vi "CRC-32.vi"(6 "Reflected":bool, 8 "FinalXorValue":u32 format="%08x", 9 "InitialCRC":u32 format="%08x", 10 "Polynomial":u32 format="%08x", 11 "DATA":u8[](array[numeric]) format="%02x") -> (3 "CRC":u32 format="%08x")   [LabVIEW 2021, in "LIN Frame Protection Addon Engine.lvlib"]
uses:
  LIN Frame Protection Addon Engine.lvlib
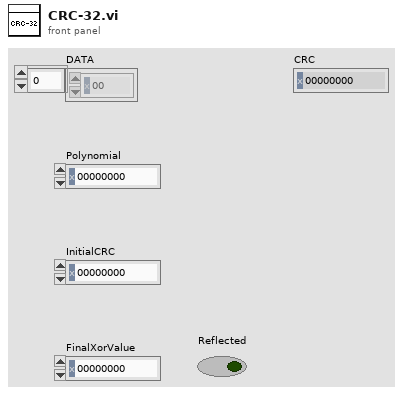
[diagram p1: front panel]
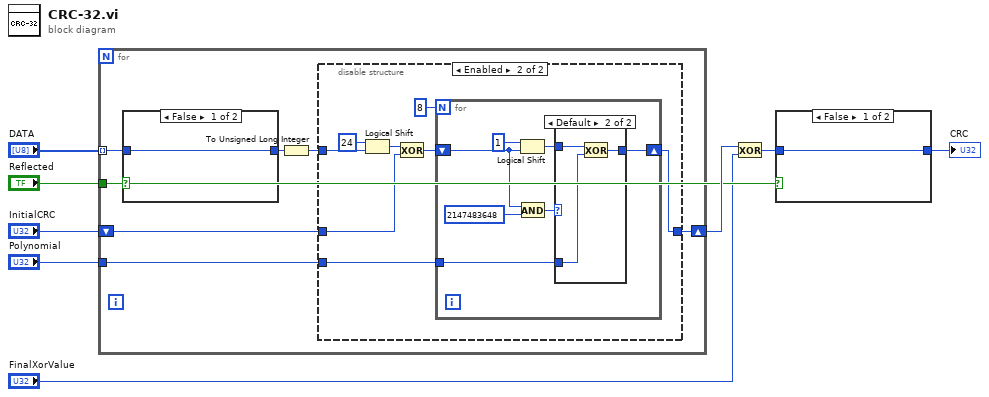
[diagram p0: block diagram]
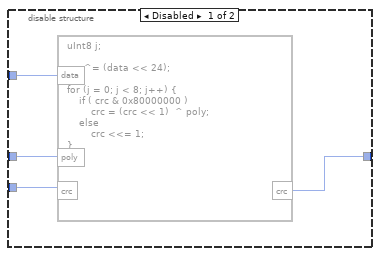
[diagram p2: hidden frame]
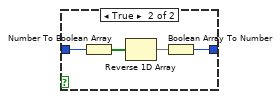
[diagram p4: hidden frame]
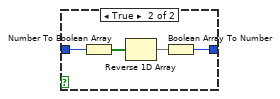
[diagram p5: hidden frame]
diagram:
  n1 = for {
    tunnel: "Polynomial" -> [w15]
    tunnel: "DATA" -> [w13] mode=indexing
    tunnel: "Reflected" -> [w14]
    shift-right: [w10] -> w6
    shift-left: "InitialCRC" -> [w11]
    n2 = case shown="False" w14 {
      tunnel: [w39 w42] -> w12
      tunnel: w13 -> [w39 w43]
      frame False {
      }
      frame True {
        n3 = Number To Boolean Array(number=w43) -> (Boolean array=w41:bool[])
        n4 = Reverse 1D Array(array=w41) -> (reversed array=w40:bool[])
        n5 = Boolean Array To Number(Boolean array=w40) -> (number=w42:u8)
      }
    }
    n6 = To Unsigned Long Integer(number=w12) -> (unsigned 32bit integer=w9:u32)
    n7 = disable-structure shown="Enabled" {
      disable-tunnel: w15 -> [w19 w22]
      disable-tunnel: w9 -> [w18 w27]
      disable-tunnel: w11 -> [w17 w25]
      disable-tunnel: [w16 w21] -> w10
      frame Disabled {
        n8 = formula code="uInt8 j;\n\ncrc ^= (data << 24);\n\nfor (j = 0; j < 8; j++) {\n    if ( crc & 0x80000000 )\n        crc = (crc << 1)  ^ poly;\n    else\n        crc <<= 1;\n}"("poly"=w19, "data"=w18, "crc"=w17) -> ("crc"=w16:u32)
      }
      frame Enabled {
        n9 = Logical Shift(y=u32 24 ("x"), x=w27) -> (x << y=w26:u32)
        n10 = Exclusive Or(1:w25, 2:w26) -> (0:w23:u32)
        n11 = for {
          N: 8 -> [_]
          tunnel: w22 -> [w29]
          shift-right: [w28] -> w21
          shift-left: w23 -> [w32]
          n12 = Logical Shift(y=i16 1, x=w32) -> (x << y=w30:u32)
          n13 = And(x=w32, y=u32 2147483648) -> (x .and. y?=w33:u32)
          n14 = case shown="Default" w33 {
            tunnel: w30 -> [w35 w38]
            tunnel: w29 -> [_ w37]
            tunnel: [w35 w36] -> w28
            frame 0 {
            }
            frame Default {
              n15 = Exclusive Or(1:w37, 2:w38) -> (0:w36:u32)
            }
          }
        }
      }
    }
  }
  n16 = Exclusive Or(1:"FinalXorValue", 2:w6) -> (0:w3:u32)
  n17 = case shown="False" "Reflected" {
    tunnel: [w44 w47] -> w4
    tunnel: w3 -> [w44 w48]
    frame False {
    }
    frame True {
      n18 = Number To Boolean Array(number=w48) -> (Boolean array=w46:bool[])
      n19 = Reverse 1D Array(array=w46) -> (reversed array=w45:bool[])
      n20 = Boolean Array To Number(Boolean array=w45) -> (number=w47:u32)
    }
  }
  "CRC" <- w4
